vi "PH_gentec_Powermeter.PC Write PSDB.vi"(0 "i ref in":refnum<vi>, 5 "error IO":errorcluster) -> (14 "i ref out":refnum<vi>, 19 "error out":errorcluster)   [LabVIEW 2014, in "PH_gentec_Powermeter.lvlib"]
doc: "This is the proc case which writes data to the PHELIX shot data base."
uses:
  PH_gentec_Powermeter.lvlib
  PH_Basics/PH_PSDBWriter/PH_PSDBWriter.lvlib
  PH_Basics/PH_Powermeter_BaseClass/PH_Powermeter_BaseClass.lvlib
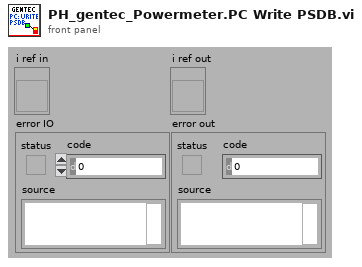
[diagram p1: front panel]
types:
  T1 = typedef "PH_Powermeter_BaseClass.lvlib/PH_Powermeter_BaseClass.i attribute.ctl" = cluster{"GUI References":T2, "Connection":T3, "Head Attributes":T5, "VISA resource":refnum<visa-resource-name>, "Energy":T6, "Service ID Energy":i32, "Wanted Settings":T7, "Current Settings":T7}
  T2 = typedef "PH_Powermeter_BaseClass.lvlib/PH_Powermeter_BaseClass.GUI Refs.ctl" = cluster{"Head Attributes":refnum<vi>, "Energy":refnum<vi>, "Connection":refnum<vi>, "VISA Resource":refnum<vi>, "Energy evolution":refnum<vi>, "Scaling Factor":refnum<vi>, "Range":refnum<vi>, "Wavelength":refnum<vi>, "Trigger Level":refnum<vi>, "Wanted Settings":refnum<vi>, "Current Settings":refnum<vi>}
  T3 = typedef "PH_Powermeter_BaseClass.lvlib/PH_Powermeter_BaseClass.Connection.ctl" = cluster{"failed checks":i8, "Timeout":bool, "Data read":string, "Failure":bool, "Error":bool, "State":T4}
  T4 = typedef "PH_Powermeter_BaseClass.lvlib/PH_Powermeter_BaseClass.State.ctl" = enum32{"off", "operating", "opened", "checked", "connected", "Sets to change", "running"}
  T5 = typedef "PH_Powermeter_BaseClass.lvlib/PH_Powermeter_BaseClass.Head Attributes.ctl" = cluster{"Instrument Type":string, "Head Version":string, "Head Name":string, "Serial Number":string, "Firmware":string, "Sensor Type":string, "MinimumRange":u32, "Maximum Range":u32, "Min Wavelength":i32, "Max Wavelength":i32}
  T6 = typedef "PH_Powermeter_BaseClass.lvlib/PH_Powermeter_BaseClass.Energy.ctl" = cluster{"current Value":dbl, "unscaled":dbl, "Scaling Factor":dbl}
  T7 = typedef "PH_Powermeter_BaseClass.lvlib/PH_gentec_BaseClass.Head Settings.ctl" = cluster{"Trigger Level":dbl, "Wavelength":u32, "Range":u32}
  T8 = typedef "PH_PSDBWriter.lvlib/PH_PSDBWriter.Numeric dataset.ctl" = cluster{"name":string, "data":dbl, "unit":string}
  T9 = typedef "PH_PSDBWriter.lvlib/PH_PSDBWriter.String dataset.ctl" = cluster{"name":string, "data":string, "unit":string}
  T10 = typedef "PH_PSDBWriter.lvlib/PH_PSDBWriter.PSDB Dataset.ctl" = cluster{"Version":i32, "2D data Input":T11[], "Boolean Input":T13[], "Image Input":T14[], "Numeric Input":T8[], "String Input":T9[]}
  T11 = typedef "PH_PSDBWriter.lvlib/PH_PSDBWriter.2D dataset.ctl" = cluster{"name":string, "data":dbl[][], "axis description":T12}
  T12 = typedef "PSDB.lvlib/PSDB_AxisDescription.ctl" = cluster{"x axis label":string, "y axis label":string, "x axis unit":string, "y axis unit":string}
  T13 = typedef "PH_PSDBWriter.lvlib/PH_PSDBWriter.Boolean dataset.ctl" = cluster{"name":string, "data":bool, "unit":string}
  T14 = typedef "PH_PSDBWriter.lvlib/PH_PSDBWriter.Image dataset.ctl" = cluster{"name":string, "data":T15, "unit":string}
  T15 = typedef "IMAQ Image.ctl" = refnum<image>
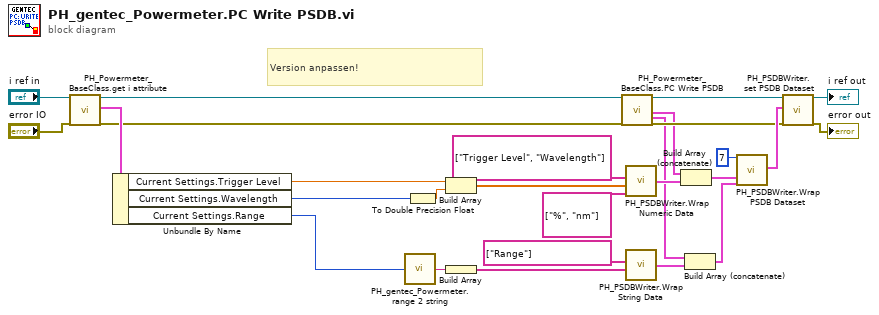
[diagram p0: block diagram]
diagram:
  # "Version anpassen!"
  n1 = call "PH_Powermeter_BaseClass.get i attribute.vi"("i ref in"="i ref in", "error in (no error)"="error IO") -> ("i ref out"=w5:refnum<vi>, "i attribute"=w27:T1, "error out"=w4:errorcluster)  [unwired: 15 in]
  n2 = Unbundle By Name(w27) -> ("Current Settings.Trigger Level"=w1:dbl, "Current Settings.Wavelength"=w26:u32, "Current Settings.Range"=w3:u32)
  n3 = call "PH_gentec_Powermeter.range 2 string.vi"("Range"=w3) -> ("Range as string"=w2:string)
  n4 = To Double Precision Float(number=w26) -> (double precision float=w25:dbl)
  n5 = Build Array(w1, w25) -> (w19:dbl[])
  n6 = Build Array(w2) -> (w15:string[])
  n7 = call "PH_Powermeter_BaseClass.PC Write PSDB.vi"("i ref in"=w5, "error IO"=w4) -> ("i ref out"=w13:refnum<vi>, "PSDB Numeric Data Array"=w8:T8[], "PSDB String Data Array"=w7:T9[], "error out"=w14:errorcluster)  [unwired: 14 in]
  n8 = call "PH_PSDBWriter.Wrap Numeric Data.vi"("Unit Array"=string[] ["%", "nm"], "Data Array"=w19, "Name Array"=string[] ["Trigger Level", "Wavelength"]) -> ("PSDB Numeric Data Array"=w18:T8[])  [unwired: 1 in]
  n9 = call "PH_PSDBWriter.Wrap String Data.vi"("Data Array"=w15, "Name Array"=string[] ["Range"]) -> ("PSDB String Data Array"=w17:T9[])  [unwired: 2 in]
  n10 = Build Array (concatenate)(w8, w18) -> (w10:T8[])
  n11 = Build Array (concatenate)(w7, w17) -> (w9:T9[])
  n12 = call "PH_PSDBWriter.Wrap PSDB Dataset.vi"("Version"=7, "Numeric Input"=w10, "String Input"=w9) -> ("PSDB Dataset"=w22:T10)  [unwired: 16 in]
  n13 = call "PH_PSDBWriter.set PSDB Dataset.vi"("VI in"=w13, "PSDB Dataset"=w22, "error in (no error)"=w14) -> ("VI out"=→"i ref out":refnum<vi>, "error out"=→"error out":errorcluster)  [unwired: 15 in]
